vi "Digilens DLP Gen2 UI .vi"(11 "TopLevel In":refnum<class "TopLevel.lvclass">) -> (3 "TopLevel Out":refnum<class "TopLevel.lvclass">)   [LabVIEW 2022 SP3, in "TopLevel.lvclass"] (continued)
        n1379 = call-dynamic "Write ConfigDict.vi"("error in (no error)"=w3787, "ConfigDIct"=w3788, "TopLevel in"=w3781) -> ("error out"=w3783:errorcluster, "TopLevel out"=w3785:refnum<class "TopLevel.lvclass">)  [unwired: 7 in]
        n1380 = Bundle By Name(cluster=w3790, "TopLevel out"=w3785) -> (w3789:T77)
      }
      frame "UI: Update Prime Config" {
        w3839 = T27 {"Interval (s)"=0.1, "PurgeDuration (s)"=0.1, "Repeats"=0, "PrimingMode"=enum."Pre-Purge", "Head"=enum."1", "Frequency (Hz)"=0, "PrintWeight"=0.1} ("PrinterMode API Data")
        n1381 = Unbundle By Name(w3888) -> ("Methods:Accessors:ConfigDict"=w3837:T16, "Prime Names.Prime 1"=w3864:string, "Prime Names.Prime 2"=w3860:string, "Prime Names.Prime 3"=w3851:string, "Prime Names.Prime 4"=w3849:string, "Prime Names.Prime 5"=w3844:string, "Prime Names.Prime 6"=w3841:string)
        n1382 = call <vilib>:"Get Dynamic CVT Data.vi"("error in (no error)"=w3836, "default value (empty variant)"=w3839, "DataName"=w3864, "dCVT DVR"=w3837) -> ("error out"=w3867:errorcluster, "value"=w3866:variant, "dCVT DVR out"=w3861:T16)  [unwired: 4 in, 1 out]
        n1383 = call <vilib>:"Get Dynamic CVT Data.vi"("default value (empty variant)"=w3839, "DataName"=w3860, "dCVT DVR"=w3861) -> ("error out"=w3862:errorcluster, "value"=w3863:variant, "dCVT DVR out"=w3856:T16)  [unwired: 5 in, 1 out]
        n1384 = call <vilib>:"Get Dynamic CVT Data.vi"("default value (empty variant)"=w3839, "DataName"=w3851, "dCVT DVR"=w3856) -> ("error out"=w3858:errorcluster, "value"=w3857:variant, "dCVT DVR out"=w3852:T16)  [unwired: 5 in, 1 out]
        n1385 = call <vilib>:"Get Dynamic CVT Data.vi"("default value (empty variant)"=w3839, "DataName"=w3849, "dCVT DVR"=w3852) -> ("error out"=w3853:errorcluster, "value"=w3854:variant, "dCVT DVR out"=w3846:T16)  [unwired: 5 in, 1 out]
        n1386 = call <vilib>:"Get Dynamic CVT Data.vi"("default value (empty variant)"=w3839, "DataName"=w3844, "dCVT DVR"=w3846) -> ("error out"=w3848:errorcluster, "value"=w3847:variant, "dCVT DVR out"=w3840:T16)  [unwired: 5 in, 1 out]
        n1387 = call <vilib>:"Get Dynamic CVT Data.vi"("default value (empty variant)"=w3839, "DataName"=w3841, "dCVT DVR"=w3840) -> ("error out"=w3842:errorcluster, "value"=w3843:variant)  [unwired: 5 in, 2 out]
        n1388 = Variant To Data(error in=w3867, type=w3839, Variant=w3866) -> (data=w3865:T27)  [unwired: 1 out]
        n1389 = Variant To Data(error in=w3862, type=w3839, Variant=w3863) -> (data=w3859:T27)  [unwired: 1 out]
        n1390 = Variant To Data(error in=w3858, type=w3839, Variant=w3857) -> (data=w3855:T27)  [unwired: 1 out]
        n1391 = Variant To Data(error in=w3853, type=w3839, Variant=w3854) -> (data=w3850:T27)  [unwired: 1 out]
        n1392 = Variant To Data(error in=w3842, type=w3839, Variant=w3843) -> (data=w3838:T27)  [unwired: 1 out]
        n1393 = Variant To Data(error in=w3848, type=w3839, Variant=w3847) -> (data=w3845:T27)  [unwired: 1 out]
        n1394 = Unbundle By Name(w3865) -> ("Interval (s)"=w3887:dbl, "PurgeDuration (s)"=w3886:dbl, "Repeats"=w3868:u8, "PrimingMode"=w3869:T13, "Frequency (Hz)"=w3831:i32)
        n1395 = Unbundle By Name(w3859) -> ("Interval (s)"=w3834:dbl, "PurgeDuration (s)"=w3835:dbl, "Repeats"=w3833:u8, "PrimingMode"=w3832:T13, "Frequency (Hz)"=w3830:i32)
        n1396 = Unbundle By Name(w3855) -> ("Interval (s)"=w3885:dbl, "PurgeDuration (s)"=w3884:dbl, "Repeats"=w3870:u8, "PrimingMode"=w3871:T13, "Frequency (Hz)"=w3829:i32)
        n1397 = Unbundle By Name(w3850) -> ("Interval (s)"=w3883:dbl, "PurgeDuration (s)"=w3882:dbl, "Repeats"=w3872:u8, "PrimingMode"=w3873:T13, "Frequency (Hz)"=w3828:i32)
        n1398 = Unbundle By Name(w3845) -> ("Interval (s)"=w3881:dbl, "PurgeDuration (s)"=w3880:dbl, "Repeats"=w3874:u8, "PrimingMode"=w3875:T13, "Frequency (Hz)"=w3827:i32)
        n1399 = Unbundle By Name(w3838) -> ("Interval (s)"=w3879:dbl, "PurgeDuration (s)"=w3878:dbl, "Repeats"=w3876:u8, "PrimingMode"=w3877:T13, "Frequency (Hz)"=w3826:i32)
        n1400 = local write "Freq 5"(w3827) -> ()
        n1401 = local write "Freq 6"(w3826) -> ()
        n1402 = local write "Prime Mode 1"(w3869) -> ()
        n1403 = local write "Freq 1"(w3831) -> ()
        n1404 = local write "Prime Mode 3"(w3871) -> ()
        n1405 = local write "Freq 3"(w3829) -> ()
        n1406 = local write "Prime Mode 4"(w3873) -> ()
        n1407 = local write "Prime Mode 5"(w3875) -> ()
        n1408 = local write "Prime Mode 6"(w3877) -> ()
        n1409 = local write "Freq 4"(w3828) -> ()
        n1410 = local write "Prime Interval 1"(w3887) -> ()
        n1411 = local write "Prime Duration 1"(w3886) -> ()
        n1412 = local write "Prime Repeats 1"(w3868) -> ()
        n1413 = local write "Prime Interval 3"(w3885) -> ()
        n1414 = local write "Prime Duration 3"(w3884) -> ()
        n1415 = local write "Prime Repeats 3"(w3870) -> ()
        n1416 = local write "Prime Interval 4"(w3883) -> ()
        n1417 = local write "Prime Duration 4"(w3882) -> ()
        n1418 = local write "Prime Repeats 4"(w3872) -> ()
        n1419 = local write "Prime Interavl 5"(w3881) -> ()
        n1420 = local write "Prime Duration 5"(w3880) -> ()
        n1421 = local write "Prime Repeats 5"(w3874) -> ()
        n1422 = local write "Prime Interval 6"(w3879) -> ()
        n1423 = local write "Prime Duration 6"(w3878) -> ()
        n1424 = local write "Prime Repeats 6"(w3876) -> ()
        n1425 = local write "Prime Duration 2"(w3835) -> ()
        n1426 = local write "Prime Interval 2"(w3834) -> ()
        n1427 = local write "Prime Mode 2"(w3832) -> ()
        n1428 = local write "Freq 2"(w3830) -> ()
        n1429 = local write "Prime Repeats 1"(w3833) -> ()
      }
      frame "UI: SetUIControlsState" {
        n1430 = Unbundle By Name(w3908) -> ()  [unwired: 1 out]
        n1431 = control-ref of="This VI"() -> (w3907:refnum<vi>)
        n1432 = To Lower Case(string=w3905) -> (all lower case string=w3903:string)
        n1433 = property class="VI"(reference=w3907) -> ("Panel"=w3906:refnum<vi>)  [unwired: 1 in, 2 out]
        n1434 = Equal?(x=w3903, y="enable") -> (x = y?=w3902:bool)
        n1435 = property class="Pnl"(reference=w3906) -> ("Controls[]"=w3893:refnum<vi>[])  [unwired: 1 in, 2 out]
        n1436 = Index Array(array=w3893) -> (element=w3897:refnum<vi>)  [unwired: 1 in]
        n1437 = Select(t=T45."Enabled" ("Disabled"), s=w3902, f=T45."Disabled and Grayed Out" ("Disabled")) -> (s? t:f=w3899:T45)
        n1438 = Type Cast(type=refnum<vi> refnum ("element"), x=w3897) -> (*(type *) &x=w3895:refnum<vi>)
        n1439 = property class="TabCtl"(reference=w3895) -> ("Pages"=w3894:refnum<vi>[])  [unwired: 1 in, 2 out]
        n1440 = for {
          tunnel: w3894 -> [w3915] mode=indexing
          tunnel: [w3914] -> w3892 mode=concatenating
          n1441 = property class="Page"(reference=w3915) -> ("Z-Order:Controls[]"=w3914:refnum<vi>[])  [unwired: 1 in, 2 out]
        }
        n1442 = for {
          tunnel: w3892 -> [w3926] mode=indexing
          tunnel: w3899 -> [w3921]
          tunnel: [w3917] -> w3898 mode=indexing
          n1443 = property class="Ctl"(reference=w3926) -> (reference out=w3924:refnum<vi>, "Label.Text"=w3917:string)  [unwired: 1 in, 1 out]
          n1444 = Equal?(x=w3917, y="IdlePrint") -> (x = y?=w3918:bool)
          n1445 = Equal?(x=w3917, y="Abort") -> (x = y?=w3919:bool)
          n1446 = Or(x=w3918, y=w3919) -> (x .or. y?=w3916:bool)
          n1447 = Select(t=T45."Enabled" ("Disabled"), s=w3916, f=w3921) -> (s? t:f=w3922:T45)
          n1448 = property class="Ctl"(reference=w3924, "DisabledEnum"=w3922) -> ()  [unwired: 1 in, 2 out]
        }
        n1449 = flat-sequence {
          tunnel: w3898 -> [_]
          frame #0 {
          }
        }
        n1450 = call <vilib>:"Add State(s) to Queue__JKI_lib_State_Machine.vi"("State(s) in (\"\")"=w3913) -> ("States Out"=w3912:string)  [unwired: 14 in]
      }
      frame "UI: Cursor Set" {
        # "Argument"
        # "Set and Unset Cursor Busy.\n(Usage: \"UI: Cursor Set >> Busy|Idle\")"
        n1451 = case shown="\"Idle\", Default" w3929 {
          tunnel: w3931 -> [w3936 w3938]
          tunnel: [w3935 w3937] -> w3930
          frame "Idle", Default {
            n1452 = call <vilib>:"Unset Busy.vi"("error in (no error)"=w3936) -> ("error out"=w3935:errorcluster)  [unwired: 10 in]
          }
          frame "Busy" {
            n1453 = call <vilib>:"Set Busy.vi"("error in (no error)"=w3938) -> ("error out"=w3937:errorcluster)  [unwired: 9 in, 1 out]
          }
        }
        n1454 = call <vilib>:"Add State(s) to Queue__JKI_lib_State_Machine.vi"("State(s) in (\"\")"=w3934) -> ("States Out"=w3933:string)  [unwired: 14 in]
      }
      frame "UI: Front Panel State" {
        # "Argument"
        # "Set Front Panel Open or Closed\n(Usage: \"UI: Front Panel State >> Open|Close\")"
        n1455 = Unbundle By Name(w3944) -> ("Core.Current VI Reference"=w3943:refnum<vi>)
        n1456 = case shown="\"Open\", Default" w3942 {
          tunnel: w3945 -> [w3951 w3964]
          tunnel: [w3953 w3965] -> w3939
          tunnel: w3943 -> [w3952 w3962]
          frame "Open", Default {
            n1457 = property class="VI"(reference=w3952, error in=w3951) -> (reference out=w3949:refnum<vi>, error out=w3950:errorcluster, "Front Panel.Open"=w3948:bool)
            n1458 = case shown="False" w3948 {
              tunnel: [w3956 w3959] -> w3953
              tunnel: w3950 -> [w3955 w3959]
              tunnel: w3949 -> [w3954 _]
              frame False {
                n1459 = invoke class="VI" method="FP.Open"(reference=w3954, error in=w3955, "Activate"=TRUE, "State"=T46."Standard") -> (error out=w3956:errorcluster)  [unwired: 1 in, 4 out]
              }
              frame True {
              }
            }
          }
          frame "Close" {
            n1460 = property class="VI"(reference=w3962, error in=w3964) -> (reference out=w3961:refnum<vi>, error out=w3963:errorcluster, "Front Panel.Open"=w3960:bool)
            n1461 = case shown="True" w3960 {
              tunnel: [w3966 w3969] -> w3965
              tunnel: w3963 -> [w3966 w3968]
              tunnel: w3961 -> [_ w3967]
              frame False {
              }
              frame True {
                n1462 = invoke class="VI" method="FP.Close"(reference=w3967, error in=w3968) -> (error out=w3969:errorcluster)  [unwired: 1 in, 2 out]
              }
            }
          }
        }
        n1463 = call <vilib>:"Add State(s) to Queue__JKI_lib_State_Machine.vi"("State(s) in (\"\")"=w3947) -> ("States Out"=w3946:string)  [unwired: 14 in]
      }
      frame "UI: Update Stage Busy" {
        n1464 = Unbundle By Name(w3981) -> ("GIS Printer"=w3980:refnum<class "GIS Printer.lvclass">, "Motor Controller"=w3979:refnum<class "Motor Controller.lvclass">, "TopLevel out"=w3973:refnum<class "TopLevel.lvclass">)
        n1465 = call-dynamic "GetStatus_TopLevel_Busy.vi"("error in (no error)"=w3971, "TopLevel in"=w3973) -> ("error out"=w3972:errorcluster, "Busy"=w3970:bool)  [unwired: 7 in, 1 out]
        n1466 = call-dynamic "GetPrinterBusy_Status_GIS Printer.vi"("error in (no error)"=w3972, "TopLevel in"=w3980) -> ("error out"=w3978:errorcluster, "Printer Busy?"=w3976:bool)  [unwired: 7 in, 1 out]
        n1467 = call "GetStageBusy_Status_MotorController.vi"("error in (no error)"=w3978, "Motor Controller in"=w3979) -> ("error out"=w3977:errorcluster, "Stage Busy?"=w3975:bool)  [unwired: 7 in, 1 out]
        n1468 = Compound Arithmetic op=OR(w3976, w3975, w3970) -> (→"Stage Busy Printer" →"Stage Busy (Stage)" →"Stage Busy (Moves)":bool)
      }
      frame "UI: Display Heater Temperature" {
        w3991 = "%#.f/%#.f" ("format string")
        n1469 = Unbundle By Name(w4004) -> ("Head Temp.Head 1.Actual"=w4003:dbl, "Head Temp.Head 1.Target"=w4002:dbl, "Head Temp.Head 2.Actual"=w4001:dbl, "Head Temp.Head 2.Target"=w4000:dbl, "Head Temp.Head 3.Actual"=w3999:dbl, "Head Temp.Head 3.Target"=w3998:dbl, "Head Temp.Head 4.Actual"=w3997:dbl, "Head Temp.Head 4.Target"=w3996:dbl, "Head Temp.Head 5.Actual"=w3995:dbl, "Head Temp.Head 5.Target"=w3994:dbl, "Head Temp.Head 6.Actual"=w3993:dbl, "Head Temp.Head 6.Target"=w3992:dbl)
        n1470 = Format Into String(format string=w3991, w4003, w4002) -> (resulting string=w3990:string)  [unwired: 2 in, 1 out]
        n1471 = Format Into String(format string=w3991, w4001, w4000) -> (resulting string=w3989:string)  [unwired: 2 in, 1 out]
        n1472 = Format Into String(format string=w3991, w3999, w3998) -> (resulting string=w3988:string)  [unwired: 2 in, 1 out]
        n1473 = Format Into String(format string=w3991, w3997, w3996) -> (resulting string=w3987:string)  [unwired: 2 in, 1 out]
        n1474 = Format Into String(format string=w3991, w3995, w3994) -> (resulting string=w3986:string)  [unwired: 2 in, 1 out]
        n1475 = Format Into String(format string=w3991, w3993, w3992) -> (resulting string=w3985:string)  [unwired: 2 in, 1 out]
        n1476 = local write "Head1 Temp 1"(w3990) -> ()
        n1477 = local write "Head2 Temp 1"(w3989) -> ()
        n1478 = local write "Head3 Temp 1"(w3988) -> ()
        n1479 = local write "Head4 Temp 1"(w3987) -> ()
        n1480 = local write "Head5 Temp 1"(w3986) -> ()
        n1481 = local write "Head6 Temp 1"(w3985) -> ()
      }
      frame "---------- Macro ----------" {
        # "Do not put any code in this frame.\n(It is a separator no-op. You can make a copy of this frame to create a new Macro frame)"
        n1482 = call <vilib>:"Add State(s) to Queue__JKI_lib_State_Machine.vi"("State(s) in (\"\")"=w4014) -> ("States Out"=w4013:string)  [unwired: 14 in]
      }
      frame "Macro: Initialize" {
        # "Initialization Macro\n(This is called once, when the VI starts)"
        n1483 = call <vilib>:"Add State(s) to Queue__JKI_lib_State_Machine.vi"("State(s) in Front (\"\")"="Data: Initialize\nData: Create Images\nInitialize Core Data\nInit: Set Jog Speed\nUI: Read Prime Config\nUI: Update Prime Config\nUI: Initialize\n/*UI: SetUIControlsState>>enable\nUI: Process Head Enabled Mode\nEvents: Register Events\nUI: Update Stage Busy\nData: Apply Persistent Data\nUI: Request Logout\nAction: Sort Recipes\nData: GetMaterialsAndColorPlanes\nData: Apply Init XML to UI\nUI: Front Panel State >> Open\nUI: PrimeHeadTimerInit\nUpdateSettings>>DAQStarted>>TRUE\nData: Read Head Status\nUI: Init Recipe Dropdowns\nUI: PrimeHeadTimerInit\nAction: Apply Process Mode>>Short Idle", "State(s) in (\"\")"=w4021) -> ("States Out"=w4020:string)  [unwired: 13 in]
      }
      frame "Macro: Exit" {
        # "Exit Macro\n(This is called once, when the VI exits)"
        n1484 = Unbundle By Name(w4028) -> ("Core.Close Panel on Exit?"=w4038:bool)
        n1485 = call <vilib>:"Clear Errors.vi"("error in (no error)"=w4026) -> ("error out"=w4023:errorcluster)  [unwired: 5 in, 1 out]
        n1486 = Unbundle By Name(w4028) -> ("Exit Event"=w4030:refnum<user-event>)
        n1487 = call <vilib>:"Add States to Queue using MultiLine String (no vData input).vi"("queue in"=w4024, "states in"="Macro: Exit", "error in"=w4023) -> ("error out"=w4022:errorcluster)  [unwired: 10 in, 2 out]
        n1488 = Generate User Event(user event=w4030, event data cluster="Exit" ("event data"), error in=w4022) -> (error out=w4027:errorcluster)  [unwired: 1 in, 1 out]
        n1489 = Select(t="UI: Front Panel State >> Close", s=w4038, f="") -> (s? t:f=w4035:string)
        n1490 = call <vilib>:"Add State(s) to Queue__JKI_lib_State_Machine.vi"("State(s) in (\"\")"=w4035, "State(s) at Back (\"\")"="Data: Update Pesrsistent Values\nUI: SetUIControlsState>>enable\nUI: Request Logout\nData: Cleanup\nEvents: Unregister Events\nExit") -> ("States Out"=w4033:string)  [unwired: 13 in]
        n1491 = call <vilib>:"Add State(s) to Queue__JKI_lib_State_Machine.vi"("State(s) in Front (\"\")"=w4033, "State(s) in (\"\")"=w4040) -> ("States Out"=w4039:string)  [unwired: 13 in]
      }
      frame "----------Events ----------" {
        # "Template Separator\n(You can make a copy of, or modify, this frame)"
      }
      frame "Events: Register Events" {
        w4055 = refnum<user-event> refnum  # TopLevel StatusChanged Event
        w4065 = refnum<user-event> refnum  # IO Status Changed Event
        w4061 = refnum<user-event> refnum  # Motor Status Changed Event
        n1492 = Unbundle By Name(w4075) -> ("Motor Controller"=w4077:refnum<class "Motor Controller.lvclass">, "IO"=w4072:refnum<class "IO.lvclass">, "GIS Printer"=w4070:refnum<class "GIS Printer.lvclass">, "TopLevel out"=w4060:refnum<class "TopLevel.lvclass">, "DLP2"=w4052:refnum<class "DLP2.lvclass">)
        n1493 = property class="DLP2.lvclass"(reference=w4052, error in=w4048) -> (error out=w4049:errorcluster, "Accessors:PublicEvents*"=w4051:T94)  [unwired: 1 out]
        n1494 = Unbundle By Name(w4051) -> ("Images"=w4050:refnum<user-event>)
        n1495 = call-dynamic "GetEvents_Motor Controller.vi"("error in (no error)"=w4049, "TopLevel in"=w4077) -> ("error out"=w4071:errorcluster, "UserEvents"=w4076:T95)  [unwired: 7 in, 1 out]
        n1496 = call-dynamic "GetEvents_IO.vi"("error in (no error)"=w4071, "TopLevel in"=w4072) -> ("error out"=w4069:errorcluster, "UserEvents"=w4073:T96)  [unwired: 7 in, 1 out]
        n1497 = Unbundle By Name(w4076) -> ("Status Changed Event"=w4062:refnum<user-event>)
        n1498 = Unbundle By Name(w4073) -> ("Status Changed Event"=w4064:refnum<user-event>)
        n1499 = call-dynamic "GetEvents_GIS Printer.vi"("error in (no error)"=w4069, "TopLevel in"=w4070) -> ("error out"=w4059:errorcluster, "UserEvents"=w4068:T97)  [unwired: 7 in, 1 out]
        n1500 = Unbundle By Name(w4068) -> ("Status Changed Event"=w4067:refnum<user-event>, "GISPollStatus"=w4080:refnum<user-event>, "GISHeadStatus"=w4081:refnum<user-event>)
        n1501 = Coerce To Type(0:w4062, 1:w4061) -> (2:w4066:refnum<user-event>)
        n1502 = call-dynamic "GetEvents_TopLevel.vi"("error in (no error)"=w4059, "TopLevel in"=w4060) -> ("error out"=w4058:errorcluster, "UserEvents"=w4057:T88)  [unwired: 7 in, 1 out]
        n1503 = Coerce To Type(0:w4064, 1:w4065) -> (2:w4063:refnum<user-event>)
        n1504 = Unbundle By Name(w4057) -> ("StatusChanged"=w4056:refnum<user-event>, "DLP GUI Config Changed"=w4053:refnum<user-event>, "Login Event"=w4047:refnum<user-event>, "HeadPrimeStatusEvent"=w4046:refnum<user-event>)
        n1505 = Coerce To Type(0:w4056, 1:w4055) -> (2:w4054:refnum<user-event>)
        n1506 = register-events(w4066, w4063, w4067, w4054, w4053, w4080, w4081, w4050, w4047, w4046) -> (reference out=w4074:refnum<event-registration>)  [unwired: 2 in, 1 out]
      }
      frame "Events: Unregister Events" {
        n1507 = Unregister For Events(event registration refnum=w4084, error in=w4082) -> (error out=w4083:errorcluster)
      }
      frame "---------Init------------" {
      }
      frame "Init: Set Jog Speed" {
        n1508 = Unbundle By Name(w4094) -> ("Motor Controller"=w4098:refnum<class "Motor Controller.lvclass">)
        n1509 = Bundle By Name(cluster=T20 {"Motor Controller Parameter"=enum."Write Speed", "value"=0} ("SetExplicitMessage API Data"), "Motor Controller Parameter"=Motor_Controller_Parameter-Set."Jog Speed", "value"=0) -> (w4104:T20)
        n1510 = Bundle By Name(cluster=T23 {"Command"=enum."GetExplicitMessage", "Arguments"="", "Data"=variant} ("API Command Cluster"), "Command"=API_Command_Enum."SetExplicitMessage", "Data"=w4104) -> (w4101:T23)
        n1511 = call-dynamic "GenerateAPIEvent_Motor Controller.vi"("error in (no error)"=w4096, "API Command Cluster"=w4101, "Motor Controller In"=w4098) -> ("error out"=w4093:errorcluster)  [unwired: 6 in, 2 out]
        n1512 = flat-sequence {
          tunnel: w4093 -> [_]
          frame #0 {
            w4107 = FALSE ("Jog (+)")
            n1513 = local write "Jog (+)"(w4107) -> ()
            n1514 = local write "Jog (-)"(w4107) -> ()
          }
        }
      }
      frame "----------DIO------------" {
      }
      frame "Initialize DO Devices" {
        # "#TODO replace with daq"
        n1515 = Unbundle By Name(w4117) -> ("IO"=w4116:refnum<class "IO.lvclass">)
        n1516 = disable-structure shown="Disabled" {
          disable-tunnel: [w4134 w4136] -> w4118
          disable-tunnel: w4116 -> [w4131 w4136]
          disable-tunnel: [w4130 w4135] -> w4115
          disable-tunnel: w4113 -> [w4129 w4135]
          frame Disabled {
            n1517 = call-dynamic "Set ICP1-DO Changed bit.vi"("error in (no error)"=w4129, "Value"=TRUE, "DO Channel"=ICP1-D0_Channel_Names."Servo ON", "IO in"=w4131) -> ("error out"=w4130:errorcluster, "IO out"=w4134:refnum<class "IO.lvclass">)  [unwired: 6 in]
          }
          frame Enabled {
          }
        }
        n1518 = disable-structure shown="Disabled" {
          disable-tunnel: w4118 -> [w4126 w4128]
          disable-tunnel: w4115 -> [w4123 w4127]
          disable-tunnel: [w4122 w4127] -> w4114
          disable-tunnel: [_ w4128] -> _
          frame Disabled {
            n1519 = call-dynamic "Set ICP1-DO Changed bit.vi"("error in (no error)"=w4123, "Value"=FALSE, "DO Channel"=ICP1-D0_Channel_Names."Clear Stage Alarm", "IO in"=w4126) -> ("error out"=w4122:errorcluster)  [unwired: 6 in, 1 out]
          }
          frame Enabled {
          }
        }
      }
      frame "----------AIO-----------" {
      }
      frame "--------Purge---------" {
      }
      frame "Prime: Send API" {
        n1520 = Unbundle By Name(w4151) -> ("TopLevel out"=w4150:refnum<class "TopLevel.lvclass">, "Pre Purge API Data"=w4149:T27)
        n1521 = call-dynamic "PrimeMode API.vi"("error in (no error)"=w4147, "Pre Purge API Data"=w4149, "TopLevel in"=w4150) -> ("error out"=w4148:errorcluster)  [unwired: 7 in, 1 out]
      }
      frame "Purge: Send API" {
        n1522 = Unbundle By Name(w4161) -> ("IO"=w4160:refnum<class "IO.lvclass">, "Purge\\PrePurge Channel Name"=w4157:T19)
        n1523 = call-dynamic "Purge PH - API.vi"("Wait (F)"=FALSE, "error in (no error)"=w4158, "Duration (s)"="Duration (s)", "ICP1-DO Channel Name"=w4157, "IO in"=w4160) -> ("error out"=w4159:errorcluster)  [unwired: 5 in, 1 out]
      }
      frame "------Pre Purge-----" {
      }
      frame "Pre Purge: Send API" {
        n1524 = Unbundle By Name(w4179) -> ("Pre Purge Parameters.No. of Repeats"=w4171:i32, "Pre Purge Parameters.GIS File Path"=w4174:path, "Pre Purge Parameters.Duration (s)"=w4173:dbl, "Purge\\PrePurge Channel Name"=w4172:T19)  [unwired: 1 out]
        n1525 = call-dynamic "Pre Purge API.vi"("Repeats"=w4171, "ICP1-DO Channel Names"=w4172, "PurgeDuration (s)"="PPDuration (s)", "error in (no error)"=w4175, "Duration (s)"=w4173, "GIS File Path"=w4174, "TopLevel in"=w4177) -> ("error out"=w4176:errorcluster, "TopLevel out"=w4178:refnum<class "TopLevel.lvclass">)  [unwired: 3 in]
      }
      frame "---------Action-------" {
      }
      frame "Action: LoadImages" {
        n1526 = case shown="\"CalibrationPrints\"" w4190 {
          tunnel: w4189 -> [_ w4204]
          tunnel: w4187 -> [w4194 w4200]
          tunnel: [w4194 w4199] -> w4188
          frame Default {
          }
          frame "CalibrationPrints" {
            n1527 = property on="PrintHead Number" class="Ring (strict)"() -> ("RingText.Text"=w4198:string)  [unwired: 2 in, 2 out]
            n1528 = Unbundle By Name(w4204) -> ("DLP2"=w4203:refnum<class "DLP2.lvclass">, "CalibrationPrints.CellPrintRecipe.CellPrint"=w4202:T81)
            n1529 = Decimal String To Number(string=w4198) -> (number=w4197:i32)  [unwired: 2 in, 1 out]
            n1530 = for {
              tunnel: w4202 -> [w4232] mode=indexing
              tunnel: [w4228] -> w4201 mode=indexing
              tunnel: w4197 -> [w4230]
              tunnel: [w4229] -> _
              tunnel: [w4228] -> w4195
              tunnel: [w4227] -> w4196
              stop <- w4227 stop-if-true
              n1531 = Unbundle By Name(w4232) -> ("#attributes.PrintImageFile"=w4231:string, "#attributes.Head"=w4229:i32)
              n1532 = Equal?(x=w4229, y=w4230) -> (x = y?=w4227:bool)
              n1533 = String To Path(string=w4231) -> (path=w4228:path)
            }
            n1534 = case shown="True" w4196 {
              tunnel: w4203 -> [_ w4217]
              tunnel: w4201 -> [_ _]
              tunnel: w4200 -> [w4205 w4214]
              tunnel: [w4205 w4213] -> w4199
              tunnel: w4195 -> [_ w4212]
              frame False {
              }
              frame True {
                n1535 = call <vilib>:"Get File Extension.vi"("file"=w4212) -> ("filename without extension"=w4211:string, "unmodified file extension"=w4210:string)  [unwired: 6 in, 3 out]
                n1536 = Strip Path(path=w4212) -> (stripped path=w4209:path)  [unwired: 1 out]
                n1537 = for {
                  N: 4 -> [_]
                  tunnel: w4211 -> [w4226]
                  tunnel: w4210 -> [w4223]
                  tunnel: w4209 -> [w4221]
                  tunnel: [w4219] -> w4207 mode=indexing
                  i -> [w4225]
                  n1538 = Number To Decimal String(number=w4225) -> (decimal integer string=w4224:string)  [unwired: 1 in]
                  n1539 = Concatenate Strings(w4226, "_" ("string"), w4224, "." ("string"), w4223) -> (w4220:string)
                  n1540 = Build Path(base path=w4221, name or relative path=w4220) -> (appended path=w4219:path)
                }
                n1541 = Bundle By Name(cluster=T47 {"Images[]"=[], "Calibration"=FALSE} ("LoadImagesData"), "Images[]"=w4207, "Calibration"=TRUE) -> (w4215:T47)
                n1542 = call "API_LoadImages.vi"("error in (no error)"=w4214, "LoadImagesData"=w4215, "DLP2 in"=w4217) -> ("error out"=w4213:errorcluster)  [unwired: 7 in, 1 out]
              }
            }
          }
        }
      }
      frame "Action: Wait for PrePrime" {
        n1543 = Unbundle By Name(w4241) -> ("PrePrimeDone"=w4240:bool)
        n1544 = Select(t="UI: EnableControls>>Print PPP Image>>True", s=w4240, f="Idle\nAction: Wait for PrePrime") -> (s? t:f=w4235:string)
        n1545 = call <userlib>:"Wait (ms)__ogtk.vi"("error in (no error)"=w4244, "milliseconds to wait"=u32 200) -> ("error out"=w4234:errorcluster)  [unwired: 8 in, 1 out]
        n1546 = call <vilib>:"Add State(s) to Queue__JKI_lib_State_Machine.vi"("State(s) in Front (\"\")"=w4235, "State(s) in (\"\")"=w4238) -> ("States Out"=w4239:string)  [unwired: 13 in]
      }
      frame "Action: PrePrimeTimer" {
        n1547 = Unbundle By Name(w4245) -> ("DAQ"=w4252:refnum<class "DAQ.lvclass">)
        n1548 = case shown="\"Check\"" w4248 {
          tunnel: [_ "Action: Wait for PrePrime"] -> w4247
          tunnel: w4245 -> [w4256 w4259]
          tunnel: [w4256 w4258] -> w4246
          frame "False", Default {
          }
          frame "Check" {
            n1549 = Bundle By Name(cluster=w4259, "PrePrimeDone"=FALSE ("PrePrimeTimerExp")) -> (w4258:T77)
          }
        }
        n1550 = call "Generate Timer Event.vi"("error in (no error)"=w4253, "CmdMsg"=w4248, "DAQ"=w4252) -> ("error out"=w4251:errorcluster)  [unwired: 7 in, 1 out]
        n1551 = call <vilib>:"Add State(s) to Queue__JKI_lib_State_Machine.vi"("State(s) in Front (\"\")"=w4247, "State(s) in (\"\")"=w4249) -> ("States Out"=w4250:string)  [unwired: 13 in]
      }
      frame "Action: Update Materials in XML" {
        n1552 = property on="Head 4 Material 2" class="Ring (strict)"(error in=w4261) -> ("RingText.Text"=w4271:string)  [unwired: 1 in, 2 out]
        n1553 = property on="Head 6 Material 2" class="Ring (strict)"(error in=w4261) -> ("RingText.Text"=w4269:string)  [unwired: 1 in, 2 out]
        n1554 = property on="Head 1 Material 2" class="Ring (strict)"(error in=w4261) -> ("RingText.Text"=w4274:string)  [unwired: 1 in, 2 out]
        n1555 = property on="Head 2 Material 2" class="Ring (strict)"(error in=w4261) -> ("RingText.Text"=w4273:string)  [unwired: 1 in, 2 out]
        n1556 = property on="Head 3 Material 2" class="Ring (strict)"(error in=w4261) -> ("RingText.Text"=w4272:string)  [unwired: 1 in, 2 out]
        n1557 = property on="Head 5 Material 2" class="Ring (strict)"(error in=w4261) -> ("RingText.Text"=w4270:string)  [unwired: 1 in, 2 out]
        n1558 = Unbundle By Name(w4278) -> ("TopLevel out"=w4279:refnum<class "TopLevel.lvclass">)
        n1559 = Build Array(w4274, w4273, w4272, w4271, w4270, w4269) -> (w4268:string[])
        n1560 = property class="TopLevel.lvclass"(reference=w4279, error in=w4261) -> (reference out=w4267:refnum<class "TopLevel.lvclass">, error out=w4263:errorcluster, "Methods:Accessors:PrinterInitializationXML"=w4277:T61)
        n1561 = Unbundle By Name(w4277) -> ("HeadSet.HeadProperties"=w4276:T63[])
        n1562 = for {
          tunnel: w4276 -> [w4290] mode=indexing
          tunnel: [w4289] -> w4275 mode=indexing
          tunnel: w4268 -> [w4288] mode=indexing
          n1563 = Bundle By Name(cluster=w4290, "#attributes.Material"=w4288) -> (w4289:T63)
        }
        n1564 = Bundle By Name(cluster=w4277, "HeadSet.HeadProperties"=w4275) -> (w4265:T61)
        n1565 = property class="TopLevel.lvclass"(reference=w4267, error in=w4263, "Methods:Accessors:PrinterInitializationXML"=w4265) -> (reference out=w4266:refnum<class "TopLevel.lvclass">, error out=w4264:errorcluster)
        n1566 = disable-structure shown="Enabled" {
          disable-tunnel: w4266 -> [w4286 _]
          disable-tunnel: w4265 -> [w4285 _]
          disable-tunnel: w4264 -> [w4284 w4287]
          disable-tunnel: [w4283 w4287] -> w4262
          frame Disabled {
            n1567 = call-dynamic "SaveInitXML_API.vi"("error in (no error)"=w4284, "InitXML"=w4285, "TopLevel in"=w4286) -> ("error out"=w4283:errorcluster)  [unwired: 7 in, 1 out]
          }
          frame Enabled {
          }
        }
      }
      frame "Action: Update PrintWeights in XML" {
        n1568 = Unbundle By Name(w4296) -> ("Methods:Accessors:ConfigDict"=w4297:T16)
        n1569 = Unbundle By Name(w4296) -> ("TopLevel out"=w4306:refnum<class "TopLevel.lvclass">, "PrintWeights"=w4298:T33)
        n1570 = Cluster To Array(cluster=w4298) -> (array=w4293:dbl[])
        n1571 = property class="TopLevel.lvclass"(reference=w4306, error in=w4295) -> (reference out=w4304:refnum<class "TopLevel.lvclass">, error out=w4300:errorcluster, "Methods:Accessors:PrinterInitializationXML"=w4305:T61)
        n1572 = Unbundle By Name(w4305) -> ("InkSet.Ink"=w4292:T65[])
        n1573 = for {
          shift-right: [w4323] -> _
          shift-left: w4297 -> [w4331]
          shift-right: [w4322] -> _
          shift-left: w4295 -> [w4330]
          tunnel: i32[] [1, 2, 3, 4, 5, 6] -> [w4320] mode=indexing
          tunnel: w4293 -> [w4316] mode=indexing
          tunnel: w4292 -> [w4319]
          tunnel: [w4315] -> w4291 mode=indexing
          w4327 = T63 {"#attributes"={"HeadNumber"=0, "Material"="", "HeadLocalX"=0.0, "HeadLocalY"=0.0, "HeadRotationAngle"=0.0, "VH2L_Hi"=0.0, "VH2R_Hi"=0.0, "VH1LA_Hi"=0.0, "VH1LB_Hi"=0.0, "VH1RA_Hi"=0.0, "VH1RB_Hi"=0.0, "VH2L_Lo"=0.0, "VH2R_Lo"=0.0, "VH1LA_Lo"=0.0, "VH1LB_Lo"=0.0, "VH1RA_Lo"=0.0, "VH1RB_Lo"=0.0}} ("HeadProperties")
          n1574 = Format Into String(w4320) -> (resulting string=w4321:string)  [unwired: 3 in, 1 out]
          n1575 = Concatenate Strings("Head " ("string"), w4321) -> (w4328:string)
          n1576 = call <vilib>:"Get Dynamic CVT Data.vi"("error in (no error)"=w4330, "default value (empty variant)"=w4327, "DataName"=w4328, "dCVT DVR"=w4331) -> ("error out"=w4325:errorcluster, "value"=w4326:variant, "dCVT DVR out"=w4323:T16)  [unwired: 4 in, 1 out]
          n1577 = Variant To Data(error in=w4325, type=w4327, Variant=w4326) -> (data=w4324:T63, error out=w4322:errorcluster)
          n1578 = Unbundle By Name(w4324) -> ("#attributes.Material"=w4318:string)
          n1579 = for {
            tunnel: w4319 -> [w4332] mode=indexing
            tunnel: w4318 -> [w4334]
            tunnel: [w4332] -> w4317
            stop <- w4333 stop-if-true
            n1580 = Unbundle By Name(w4332) -> ("#attributes.InkType"=w4335:string)
            n1581 = Equal?(x=w4335, y=w4334) -> (x = y?=w4333:bool)
          }
          n1582 = Bundle By Name(cluster=w4317, "#attributes.PrintWeight"=w4316) -> (w4315:T65)
        }
        n1583 = Bundle By Name(cluster=w4305, "InkSet.Ink"=w4291) -> (w4302:T61)
        n1584 = property class="TopLevel.lvclass"(reference=w4304, error in=w4300, "Methods:Accessors:PrinterInitializationXML"=w4302) -> (reference out=w4303:refnum<class "TopLevel.lvclass">, error out=w4301:errorcluster)
        n1585 = disable-structure shown="Enabled" {
          disable-tunnel: w4303 -> [w4313 _]
          disable-tunnel: w4302 -> [w4312 _]
          disable-tunnel: w4301 -> [w4311 w4314]
          disable-tunnel: [w4310 w4314] -> w4299
          frame Disabled {
            n1586 = call-dynamic "SaveInitXML_API.vi"("error in (no error)"=w4311, "InitXML"=w4312, "TopLevel in"=w4313) -> ("error out"=w4310:errorcluster)  [unwired: 7 in, 1 out]
          }
          frame Enabled {
          }
        }
      }
      frame "Action: Update MeniscusPressure in XML" {
        n1587 = Unbundle By Name(w4348) -> ("Methods:Accessors:ConfigDict"=w4349:T16)
        n1588 = property on="Meniscus Pressure Set - R6" class="DigNum (strict)"() -> ("Value"=w4338:dbl)  [unwired: 2 in, 2 out]
        n1589 = property on="Meniscus Pressure Set - R4" class="DigNum (strict)"() -> ("Value"=w4340:dbl)  [unwired: 2 in, 2 out]
        n1590 = property on="Meniscus Pressure Set - R5" class="DigNum (strict)"() -> ("Value"=w4339:dbl)  [unwired: 2 in, 2 out]
        n1591 = property on="Meniscus Pressure Set - R2" class="DigNum (strict)"() -> ("Value"=w4342:dbl)  [unwired: 2 in, 2 out]
        n1592 = property on="Meniscus Pressure Set - R3" class="DigNum (strict)"() -> ("Value"=w4341:dbl)  [unwired: 2 in, 2 out]
        n1593 = property on="Meniscus Pressure Set - R1" class="DigNum (strict)"() -> ("Value"=w4343:dbl)  [unwired: 2 in, 2 out]
        n1594 = Unbundle By Name(w4348) -> ("TopLevel out"=w4357:refnum<class "TopLevel.lvclass">)
        n1595 = Build Array(w4343, w4342, w4341, w4340, w4339, w4338) -> (w4337:dbl[])
        n1596 = property class="TopLevel.lvclass"(reference=w4357, error in=w4347) -> (reference out=w4355:refnum<class "TopLevel.lvclass">, error out=w4351:errorcluster, "Methods:Accessors:PrinterInitializationXML"=w4356:T61, "Methods:Accessors:ProcessMode"=w4336:T9)
        n1597 = Unbundle By Name(w4356) -> ("InkSet.Ink"=w4345:T65[])
        n1598 = for {
          shift-right: [w4375] -> _
          shift-left: w4349 -> [w4383]
          shift-right: [w4374] -> _
          shift-left: w4347 -> [w4382]
          tunnel: i32[] [1, 2, 3, 4, 5, 6] -> [w4372] mode=indexing
          tunnel: w4337 -> [w4368] mode=indexing
          tunnel: w4345 -> [w4371]
          tunnel: [w4367] -> w4344 mode=indexing
          tunnel: w4336 -> [w4366]
          w4379 = T63 {"#attributes"={"HeadNumber"=0, "Material"="", "HeadLocalX"=0.0, "HeadLocalY"=0.0, "HeadRotationAngle"=0.0, "VH2L_Hi"=0.0, "VH2R_Hi"=0.0, "VH1LA_Hi"=0.0, "VH1LB_Hi"=0.0, "VH1RA_Hi"=0.0, "VH1RB_Hi"=0.0, "VH2L_Lo"=0.0, "VH2R_Lo"=0.0, "VH1LA_Lo"=0.0, "VH1LB_Lo"=0.0, "VH1RA_Lo"=0.0, "VH1RB_Lo"=0.0}} ("HeadProperties")
          n1599 = Format Into String(w4372) -> (resulting string=w4373:string)  [unwired: 3 in, 1 out]
          n1600 = Concatenate Strings("Head " ("string"), w4373) -> (w4380:string)
          n1601 = call <vilib>:"Get Dynamic CVT Data.vi"("error in (no error)"=w4382, "default value (empty variant)"=w4379, "DataName"=w4380, "dCVT DVR"=w4383) -> ("error out"=w4377:errorcluster, "value"=w4378:variant, "dCVT DVR out"=w4375:T16)  [unwired: 4 in, 1 out]
          n1602 = Variant To Data(error in=w4377, type=w4379, Variant=w4378) -> (data=w4376:T63, error out=w4374:errorcluster)
          n1603 = Unbundle By Name(w4376) -> ("#attributes.Material"=w4370:string)
          n1604 = for {
            tunnel: w4371 -> [w4393] mode=indexing
            tunnel: w4370 -> [w4395]
            tunnel: [w4393] -> w4369
            stop <- w4394 stop-if-true
            n1605 = Unbundle By Name(w4393) -> ("#attributes.InkType"=w4396:string)
            n1606 = Equal?(x=w4396, y=w4395) -> (x = y?=w4394:bool)
          }
          n1607 = case shown="\"Process\"" w4366 {
            tunnel: w4369 -> [w4386 w4389 w4392]
            tunnel: w4368 -> [w4384 w4387 w4391]
            tunnel: [w4385 w4388 w4390] -> w4367
            frame "Short Idle", Default {
              n1608 = Bundle By Name(cluster=w4386, "Idle.ShortIdle.#attributes.Meniscus"=w4384) -> (w4385:T65)
            }
            frame "Process" {
              n1609 = Bundle By Name(cluster=w4389, "#attributes.Meniscus"=w4387) -> (w4388:T65)
            }
            frame "Long Idle " {
              n1610 = Bundle By Name(cluster=w4392, "Idle.LongIdle.#attributes.Meniscus"=w4391) -> (w4390:T65)
            }
          }
        }
        n1611 = Bundle By Name(cluster=w4356, "InkSet.Ink"=w4344) -> (w4353:T61)
        n1612 = property class="TopLevel.lvclass"(reference=w4355, error in=w4351, "Methods:Accessors:PrinterInitializationXML"=w4353) -> (reference out=w4354:refnum<class "TopLevel.lvclass">, error out=w4352:errorcluster)
        n1613 = disable-structure shown="Enabled" {
          disable-tunnel: w4354 -> [w4364 _]
          disable-tunnel: w4353 -> [w4363 _]
          disable-tunnel: w4352 -> [w4362 w4365]
          disable-tunnel: [w4361 w4365] -> w4350
          frame Disabled {
            n1614 = call-dynamic "SaveInitXML_API.vi"("error in (no error)"=w4362, "InitXML"=w4363, "TopLevel in"=w4364) -> ("error out"=w4361:errorcluster)  [unwired: 7 in, 1 out]
          }
          frame Enabled {
          }
        }
      }
      frame "Action: Update INI XML" {
        n1615 = Unbundle By Name(w4399) -> ("TopLevel out"=w4400:refnum<class "TopLevel.lvclass">)
        n1616 = property class="TopLevel.lvclass"(reference=w4400) -> (reference out=w4401:refnum<class "TopLevel.lvclass">, "Methods:Accessors:PrinterInitializationXML"=w4402:T61)  [unwired: 1 in, 1 out]
        n1617 = call-dynamic "SaveInitXML_API.vi"("error in (no error)"=w4397, "InitXML"=w4402, "TopLevel in"=w4401) -> ("error out"=w4398:errorcluster)  [unwired: 7 in, 1 out]
      }
      frame "Action: Print Head" {
      }
      frame "Action: Apply Process Mode" {
        w4447 = T18[] [enum."1", enum."2", enum."3", enum."4", enum."5", enum."6"] items=["-1", "1", "2", "3", "4", "5", "6"] ("Heater Enable.Head")
        n1618 = Unbundle By Name(w4445) -> ("TopLevel out"=w4444:refnum<class "TopLevel.lvclass">)
        n1619 = property class="TopLevel.lvclass"(reference=w4444, error in=w4440) -> (reference out=w4415:refnum<class "TopLevel.lvclass">, error out=w4413:errorcluster, "Methods:Accessors:PrinterInitializationXML"=w4446:T61, "Methods:Accessors:ConfigDict"=w4433:T16)
        n1620 = Unbundle By Name(w4446) -> ("PrinterInitialization.HIBEnable.#attributes"=w4411:T98, "InkSet.Ink"=w4432:T65[])
        n1621 = call "GetProcessModeParamsFromDict.vi"("PrinterInitialization.HIBEnable.#attributes"=w4411, "Ink"=w4432, "Data Value Reference in"=w4433) -> ("ProcessModeParams"=w4429:T99)  [unwired: 8 in]
        n1622 = Unbundle By Name(w4429) -> ("Head Array"=w4425:u8[], "ProcessHeat[]"=w4428:dbl[], "ShortIdleHeat[]"=w4427:dbl[], "LongIdleHeat[]"=w4426:dbl[], "ProcessMeniscus[]"=w4424:dbl[], "ShortIdleMeniscus[]"=w4423:dbl[], "LongIdleMeniscus[]"=w4422:dbl[], "ProcessRecirc[]"=w4421:bool[], "ShortIdleRecirc[]"=w4420:bool[], "LongIdleRecirc[]"=w4419:bool[])
        n1623 = case shown="\"Short Idle\", Default" w4430 {
          tunnel: w4426 -> [_ w4457 _]
          tunnel: w4427 -> [w4453 _ _]
          tunnel: w4428 -> [_ _ w4461]
          tunnel: [w4453 w4457 w4461] -> w4431
          tunnel: [processMode--enum."Short Idle" ("ProcessMode") processMode--enum."Long Idle " ("ProcessMode") processMode--enum."Process" ("ProcessMode")] -> w4416
          tunnel: w4424 -> [_ _ w4459]
          tunnel: w4423 -> [w4451 _ _]
          tunnel: w4422 -> [_ w4455 _]
          tunnel: w4421 -> [_ _ w4458]
          tunnel: w4420 -> [w4450 _ _]
          tunnel: w4419 -> [_ w4454 _]
          tunnel: [w4451 w4455 w4459] -> w4418
          tunnel: [w4450 w4454 w4458] -> w4417
          frame "Short Idle", Default {
          }
          frame "Long Idle" {
          }
          frame "Process" {
          }
        }
        n1624 = Cluster To Array(cluster=w4411) -> (array=w4443:bool[])
        n1625 = local write "ProcessMode"(w4416) -> ()
        n1626 = call-dynamic "Write ProcessMode.vi"("error in (no error)"=w4413, "ProcessMode"=w4416, "TopLevel in"=w4415) -> ("error out"=w4412:errorcluster, "TopLevel out"=w4414:refnum<class "TopLevel.lvclass">)  [unwired: 7 in]
        n1627 = for {
          tunnel: w4425 -> [w4484] mode=indexing
          tunnel: [w4483] -> w4437 mode=indexing
          shift-right: [w4481] -> w4442
          shift-left: w4412 -> [w4482]
          tunnel: w4443 -> [w4480] mode=indexing
          tunnel: w4431 -> [w4479] mode=indexing
          tunnel: w4418 -> [w4478] mode=indexing
          tunnel: w4417 -> [w4477] mode=indexing
          n1628 = case shown="True" w4480 {
            tunnel: w4484 -> [_ w4487]
            tunnel: [_ w4492] -> w4483
            tunnel: w4482 -> [w4485 w4491]
            tunnel: [w4485 w4490] -> w4481
            tunnel: w4479 -> [_ w4489]
            tunnel: w4478 -> [_ w4488]
            tunnel: w4477 -> [_ w4486]
            frame False {
            }
            frame True {
              n1629 = Format Into String(format string="Set Head Temperature>>%d>>%f\nSet Meniscus Pressure Value>>%d>>%f\nSetRecircPump>>%d>>%s", error in=w4491, w4487, w4489, w4487, w4488, w4487, w4486) -> (resulting string=w4492:string, error out=w4490:errorcluster)  [unwired: 1 in]
            }
          }
        }
        n1630 = Array To Spreadsheet String(delimiter (Tab)="\n", array=w4437, 3:"" ("format string")) -> (spreadsheet string=w4434:string)
        n1631 = for {
          shift-right: [w4466] -> _
          shift-left: w4414 -> [w4467]
          shift-right: [w4464] -> w4441
          shift-left: w4442 -> [w4465]
          tunnel: w4447 -> [w4463] mode=indexing
          tunnel: w4443 -> [w4462] mode=indexing
          n1632 = case shown="True" w4462 {
            tunnel: w4467 -> [w4469 w4476]
            tunnel: [w4469 w4475] -> w4466
            tunnel: w4465 -> [w4468 w4474]
            tunnel: [w4468 w4473] -> w4464
            tunnel: w4463 -> [_ w4472]
            tunnel: w4462 -> [_ w4471]
            frame False {
            }
            frame True {
              n1633 = call-dynamic "EnableHeadHeater API.vi"("Wait (F)"=TRUE, "error in (no error)"=w4474, "Enable"=w4471, "Head"=w4472, "TopLevel in"=w4476) -> ("error out"=w4473:errorcluster, "TopLevel out"=w4475:refnum<class "TopLevel.lvclass">)  [unwired: 5 in]
            }
          }
        }
        n1634 = call <vilib>:"Add State(s) to Queue__JKI_lib_State_Machine.vi"("State(s) in Front (\"\")"=w4434, "State(s) in (\"\")"=w4438) -> ("States Out"=w4439:string)  [unwired: 13 in]
      }
      frame "Action: Sort Recipes" {
        w4505 = T100 {"Products"=[], "RecipeTypes"=[]}
        n1635 = Unbundle By Name(w4511) -> ("TopLevel out"=w4510:refnum<class "TopLevel.lvclass">)  [unwired: 1 out]
        n1636 = call "FG - FilePathnames.vi"() -> ("FilePaths out"=w4495:T83)  [unwired: 4 in, 1 out]
        n1637 = Unbundle By Name(w4495) -> ("RecipeXMLFolder"=w4494:path)
        n1638 = call "Sortrecipestypes.vi"("error in (no error)"=w4508, "RecipeFolderPath"=w4494, "TopLevel.lvclass"=w4510) -> ("error out"=w4497:errorcluster, "reference out"=w4502:refnum<class "TopLevel.lvclass">)  [unwired: 4 in, 3 out]
        n1639 = property class="TopLevel.lvclass"(reference=w4502) -> (reference out=w4501:refnum<class "TopLevel.lvclass">, "Methods:Accessors:ConfigDict"=w4500:T16)  [unwired: 1 in, 1 out]
        n1640 = call <vilib>:"Get Dynamic CVT Data.vi"("error in (no error)"=w4497, "default value (empty variant)"=w4505, "DataName"="RecipesSummary", "dCVT DVR"=w4500) -> ("error out"=w4504:errorcluster, "value"=w4506:variant)  [unwired: 4 in, 2 out]
        n1641 = Variant To Data(error in=w4504, type=w4505, Variant=w4506) -> (data=w4503:T100, error out=w4498:errorcluster)
        n1642 = Bundle By Name(cluster=w4511, "TopLevel out"=w4501) -> (w4509:T77)
        n1643 = Unbundle By Name(w4503) -> ("RecipeTypes"=w4499:string[])
        n1644 = property on="RecipeType" class="Ring (strict)"(error in=w4498, "Strings []"=w4499) -> (error out=w4496:errorcluster)  [unwired: 1 in, 1 out]
      }
      frame "Action: Load Print Design" {
        n1645 = Unbundle By Name(w4518) -> ("Print.RecipeXMLPath"=w4517:path)
        n1646 = call "DLP_RecipePrints_XML_Read.vi"("error in (no error)"=w4515, "Recipe XML File Path"=w4517) -> ("error out"=w4516:errorcluster)  [unwired: 8 in, 1 out]
      }
      frame "Action: Load Calibration Prints" {
        n1647 = Unbundle By Name(w4525) -> ("Print.RecipeXMLPath"=w4524:path)
        n1648 = call "DLP_CalibrationPrints_XML_Read.vi"("error in (no error)"=w4523, "Recipe XML File Path"=w4524) -> ("error out"=w4522:errorcluster)  [unwired: 8 in, 1 out]
      }
      frame "Action: Separate Layers" {
        (unwired) 360 ("DPI_x")
        # "This case is only called for Print Design recipes"
        n1649 = Unbundle By Name(w4557) -> ("DLP2"=w4555:refnum<class "DLP2.lvclass">, "PrintDesign.Path"=w4546:path)
        n1650 = call "DLP_RecipePrints_XML_Read.vi"("error in (no error)"=w4544, "Recipe XML File Path"=w4546) -> ("error out"=w4545:errorcluster, "DLPRecipe"=w4543:T73)  [unwired: 8 in]
        n1651 = Unbundle By Name(w4543) -> ("CellPrintRecipe.CellPrint"=w4542:T92)
        n1652 = Index Array(array=w4542) -> (element=w4541:T93)  [unwired: 1 in]
        n1653 = Unbundle By Name(w4541) -> ("#attributes.PrintImageFile"=w4539:string, "#attributes.PrintMode"=w4535:string)
        n1654 = call "GetDPIValuesFromMode.vi"("PrintMode"=w4535) -> ("y"=w4533:i32, "x"=w4534:i32)  [unwired: 7 in, 2 out]
        n1655 = String To Path(string=w4539) -> (path=w4540:path)
        n1656 = Strip Path(path=w4540) -> (stripped path=w4552:path)  [unwired: 1 out]
        n1657 = call <vilib>:"Get File Extension.vi"("error in (no error)"=w4545, "file"=w4540) -> ("error out"=w4549:errorcluster, "filename without extension"=w4551:string)  [unwired: 5 in, 3 out]
        n1658 = Build Path(base path=w4552, name or relative path=w4551) -> (appended path=w4550:path)
        n1659 = call <userlib>:"Create Dir if Non-Existant__ogtk.vi"("error in (no error)"=w4549, "Directory Path"=w4550) -> ("error out"=w4548:errorcluster, "dup Directory Path"=w4547:path)  [unwired: 7 in, 1 out]
        n1660 = Bundle By Name(cluster=T49 {"Path_to_Tiff"=path "", "OutputFolder"=path "", "DPI_x"=0, "DPI_y"=0, "Python_Version"=enum."3.9 32"}, "Path_to_Tiff"=w4540, "OutputFolder"=w4547, "DPI_x"=w4534, "DPI_y"=w4533, "Python_Version"=PythonVersion--Enum."3.12 64") -> (w4537:T49)
        n1661 = call "API_SeperateLayersPython.vi"("Timeout (ms)"=u32 10000, "Wait (F)"=TRUE, "error in (no error)"=w4548, 10:w4537, "DLP2 in"=w4555) -> ("error out"=w4532:errorcluster)  [unwired: 4 in, 2 out]
        n1662 = case shown="No Error" w4532 {
          tunnel: ["UI: EnableControls>>SeparateLayers>>False" ("DictName") _] -> w4529
          frame No Error {
          }
          frame Error {
          }
        }
        n1663 = Bundle By Name(cluster=w4557, "SeparateLayers"=w4537) -> (w4538:T77)
        n1664 = call <vilib>:"Add State(s) to Queue__JKI_lib_State_Machine.vi"("State(s) in Front (\"\")"=w4529, "State(s) in (\"\")"=w4530) -> ("States Out"=w4531:string)  [unwired: 13 in]
      }
      frame "Action: Print PPP Image" {
        w4581 = "_" ("string")
        # "<Date Code>_<Product>_<Printer Name>_*.bmp"
        # "<Date Code>_<Project>_<DOE####>_<Printer Name>_<Printhead #>_<Ink Type>.bmp"
        n1665 = Unbundle By Name(w4582) -> ("TopLevel out"=w4583:refnum<class "TopLevel.lvclass">, "PPP_Ditherered_Images"=w4570:path[])
        n1666 = Unbundle By Name(w4582) -> ("PrintDesign.Path"=w4589:path)
        n1667 = call "DLP_RecipePrints_XML_Read.vi"("Recipe XML File Path"=w4589) -> ("DLPRecipe"=w4588:T73)  [unwired: 9 in, 1 out]
        n1668 = property class="TopLevel.lvclass"(reference=w4583) -> (reference out=w4573:refnum<class "TopLevel.lvclass">, "Methods:Accessors:PrinterInitializationXML"=w4584:T61)  [unwired: 1 in, 1 out]
        n1669 = Unbundle By Name(w4588) -> ("CellPrintRecipe.#attributes.Product"=w4585:string)  [unwired: 1 out]
        n1670 = Unbundle By Name(w4584) -> ("PrinterInitialization.Printer.#attributes.Name"=w4580:string)
        n1671 = Get Date/Time In Seconds() -> (seconds since 1Jan1904=w4587:timestamp)
        n1672 = Format Date/Time String(time format string (%c)="%Y%m%d_%H%M", seconds (now)=w4587) -> (date/time string=w4586:string)  [unwired: 1 in]
        "date/time string" <- w4586
        n1673 = Array Size(array=w4570) -> (size(s)=w4571:i32)
        n1674 = In Range and Coerce(upper limit=6, x=w4571, lower limit=4) -> (In Range?=w4576:bool)  [unwired: 1 out]
        n1675 = Concatenate Strings(w4586, w4581, w4585, w4581, w4580) -> (w4575:string)
        "PPP search string" <- w4575
        n1676 = case shown="True" w4576 {
          selector: w4576 -> [w4601 w4603]
          tunnel: w4570 -> [_ w4608]
          tunnel: w4575 -> [_ w4607]
          tunnel: [w4602 w4606] -> w4565
          tunnel: w4579 -> [w4602 w4605]
          tunnel: [_ w4604] -> w4574
          tunnel: [w4601 w4603] -> w4563
          frame False {
          }
          frame True {
            n1677 = for {
              tunnel: w4608 -> [w4611] mode=indexing
              tunnel: w4607 -> [w4612]
              shift-right: [w4609] -> w4606
              shift-left: w4605 -> [w4610]
              tunnel: [w4614] -> w4604
              i -> [w4613]
              n1678 = call "PrepDitheredImageNamesForPrinting.vi"("error in (no error)"=w4610, "String"=w4612, "Iteration"=w4613, "PPP_Dithered_Images"=w4611) -> ("error out"=w4609:errorcluster, "appended path"=w4614:path)  [unwired: 6 in]
            }
          }
        }
        n1679 = Unbundle By Name(w4565) -> ("status"=w4564:bool)
        n1680 = Not(x=w4564) -> (.not. x?=w4562:bool)
        n1681 = And(x=w4563, y=w4562) -> (x .and. y?=w4561:bool)
        n1682 = case shown="True" w4561 {
          tunnel: w4574 -> [_ w4599]
          tunnel: w4573 -> [_ w4598]
          tunnel: w4565 -> [w4593 w4595]
          tunnel: [w4593 w4597] -> w4572
          tunnel: ["UI: Update Status>>PPP Image Print Command NOT Executed. Did not find all Images" ("format string") _] -> w4566
          frame False {
          }
          frame True {
            n1683 = Format Into String(format string="P,C,P,\"Print Manager,Print Line Manager,PMB,PrintGoSource\",\"TTL\"\nP,C,P,\"Print Manager,Print Line Manager,PMB,EncoderSource\",\"RS422\"\nP,P,1,%s,1", error in=w4595, w4599) -> (resulting string=w4596:string, error out=w4594:errorcluster)  [unwired: 1 in]
            n1684 = call-dynamic "SendPrinterString API.vi"("error in (no error)"=w4594, "Printer String"=w4596, "TopLevel in"=w4598) -> ("error out"=w4597:errorcluster)  [unwired: 7 in, 1 out]
          }
        }
        n1685 = call <vilib>:"Add State(s) to Queue__JKI_lib_State_Machine.vi"("State(s) in Front (\"\")"=w4566, "State(s) in (\"\")"=w4567) -> ("States Out"=w4568:string)  [unwired: 13 in]
      }
      frame "Action: Invoke PPP" {
        # "To build the PPP cluster\n1. Get Material for each layer\n2. use material Name to get corresponding head no\n2a. Use Material Name to get properties for that material from dict\n3. Use Head No to get properties for that head from dict\n4. use material Name to get Material/ink compensation from Rx\n5. Get Printer properties from init xml"
        n1686 = call "BuildCommand_InvokePPP.vi"("error in (no error)"=w4621, "Cluster"=w4622) -> ("error out"=w4615:errorcluster, "NextState"=w4618:string, "PPP Dithered Images"=w4616:path[])  [unwired: 7 in]
        n1687 = Bundle By Name(cluster=w4622, "PPP_Ditherered_Images"=w4616) -> (w4617:T77)
        n1688 = call <vilib>:"Add State(s) to Queue__JKI_lib_State_Machine.vi"("State(s) in Front (\"\")"=w4618, "State(s) in (\"\")"=w4619) -> ("States Out"=w4620:string)  [unwired: 13 in]
      }
      frame "Action: Planes to RGB Image" {
        n1689 = Unbundle By Name(w4657) -> ("Planes Image"=w4635:T6, "RGB Image"=w4648:T6, "TIFFImageData.ImageBufferMain"=w4656:u8[][])
        n1690 = for {
          tunnel: w4656 -> [w4671] mode=indexing
          tunnel: [w4670] -> w4649 mode=indexing
          tunnel: [w4669] -> w4655 mode=indexing
          tunnel: [w4668] -> w4654 mode=indexing
          tunnel: [w4667] -> w4653 mode=indexing
          tunnel: [w4666] -> w4652 mode=indexing
          tunnel: [w4665] -> w4651 mode=indexing
          tunnel: [w4664] -> w4650 mode=indexing
          n1691 = Decimate 1D Array(w4671) -> (w4669:u8[], w4668:u8[], w4667:u8[], w4666:u8[], w4665:u8[], w4664:u8[])
          n1692 = for {
            tunnel: w4669 -> [w4675] mode=indexing
            tunnel: w4668 -> [w4674] mode=indexing
            tunnel: w4667 -> [w4673] mode=indexing
            tunnel: w4666 -> [w4672] mode=indexing
            tunnel: [w4676] -> w4670 mode=indexing
            tunnel: w4665 -> [_] mode=indexing
            tunnel: w4664 -> [_] mode=indexing
            n1693 = formula code="int R=255*(1-C)*(1-K);\nint G=255*(1-M)*(1-K);\nint B=255*(1-Y)*(1-K);"("C"=w4675, "Y"=w4674, "M"=w4673, "K"=w4672) -> ("R"=w4679:i32, "G"=w4678:i32, "B"=w4677:i32)
            n1694 = call <vilib>:"RGB to Color.vi"("B"=w4677, "G"=w4678, "R"=w4679) -> ("Color"=w4676:u32)
          }
        }
        n1695 = Transpose 2D Array(2D array=w4649) -> (transposed array=w4647:u32[][])
        n1696 = Bundle(w4655) -> (w4645:cluster{u8[][]})  [unwired: 1 in]
        n1697 = Bundle(w4654) -> (w4644:cluster{u8[][]})  [unwired: 1 in]
        n1698 = Bundle(w4653) -> (w4643:cluster{u8[][]})  [unwired: 1 in]
        n1699 = Bundle(w4652) -> (w4642:cluster{u8[][]})  [unwired: 1 in]
        n1700 = Bundle(w4651) -> (w4641:cluster{u8[][]})  [unwired: 1 in]
        n1701 = Bundle(w4650) -> (w4640:cluster{u8[][]})  [unwired: 1 in]
        n1702 = Build Array(w4645, w4644, w4643, w4642, w4641, w4640) -> (w4639:cluster{u8[][]}[])
        n1703 = call "IMAQ ArrayToColorImage"("Image Pixels (U32)"=w4647, "Image"=w4648, "error in (no error)"=w4646) -> ("Image Out"=w4633:T6, "error out"=w4636:errorcluster)  [unwired: 2 in]
        n1704 = for {
          tunnel: w4639 -> [w4663] mode=indexing
          tunnel: [w4661] -> w4637 mode=concatenating
          n1705 = Unbundle(w4663) -> (w4662:u8[][])
          n1706 = Transpose 2D Array(2D array=w4662) -> (transposed array=w4661:u8[][])
        }
        n1707 = call "IMAQ ArrayToImage"("error in (no error)"=w4636, "Image Pixels (U8)"=w4637, "Image"=w4635) -> ("error out"=w4631:errorcluster, "Image Out"=w4634:T6)  [unwired: 7 in]
        n1708 = Select(t=w4633, s=FALSE, f=w4634) -> (s? t:f=w4632:T6)
        "ImageMain" <- w4632
        n1709 = call "IMAQ GetImageSize"("Image"=w4632, "error in (no error)"=w4631) -> ("Y Resolution"=w4628:i32, "X Resolution"=w4627:i32, "error out"=w4630:errorcluster)  [unwired: 2 in]
        n1710 = Bundle By Name(cluster=T34 {"X Resolution"=0, "Y Resolution"=0} ("Image Resolution"), "X Resolution"=w4627, "Y Resolution"=w4628) -> (w4626:T34)
        n1711 = Bundle By Name(cluster=w4657, "RGB Image"=w4633, "Planes Image"=w4634, "Image Resolution"=w4626) -> (w4638:T77)
      }
      frame "Ink: Send Enable Command" {
        n1712 = Unbundle By Name(w4681) -> ("API Command"=w4680:T26)
        n1713 = Bundle By Name(cluster=T29 {"Command"=enum."Execute Printer Commands", "Arguments"="", "Data"=variant} ("API Command Cluster"), "Command"=w4680) -> (w4682:T29)
        n1714 = call-dynamic "GenerateAPIEvent_TopLevel.vi"("error in (no error)"=w4684, "API Command Cluster"=w4682, "TopLevel in"=w4686) -> ("error out"=w4685:errorcluster, "TopLevel out"=w4687:refnum<class "TopLevel.lvclass">)  [unwired: 7 in]
      }
      frame "------------Head Heater------------" {
      }
      frame "Heater: Enable Disable" {
        n1715 = Unbundle By Name(w4700) -> ("TopLevel out"=w4699:refnum<class "TopLevel.lvclass">, "Heater Enable.HeaterEnblHead"=w4698:T18, "Heater Enable.Enable"=w4697:bool)
        n1716 = call-dynamic "EnableHeadHeater API.vi"("error in (no error)"=w4695, "Enable"=w4697, "Head"=w4698, "TopLevel in"=w4699) -> ("error out"=w4696:errorcluster)  [unwired: 6 in, 1 out]
      }
      frame "---------Vacuum Pump----------" {
      }
      frame "Set Vacuum Pump Speed" {
        n1717 = Unbundle By Name(w4716) -> ("DAQ"=w4720:refnum<class "DAQ.lvclass">)
